vi "New User.vi"() -> ()   [LabVIEW 2020, in "User Lib.lvlib"]
uses:
  User Lib.lvlib
  <vilib>/addons/database/Connection.llb/DB Tools Open Connec (String).vi
  <vilib>/addons/database/_DB Variant To Data/Database Variant To Data.xnode
  <vilib>/addons/database/NI_Database_API.lvlib
  Database Lib.lvlib
panel:
  out "Error out":errorcluster
  out "Error out 2":errorcluster
  in  "Cancel":bool
  in  "OK":bool
  in  "Is Admin?":enum32{"Yes", "No"}(radio)
  in  "Full Name":string
  in  "Confirm Password":string
  in  "Password":string
  in  "Username":string
  # "New User"
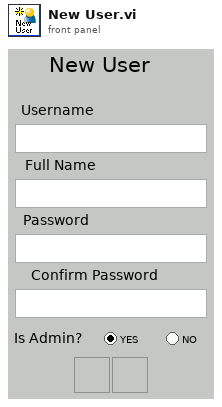
[diagram p1: front panel]
types:
  T1 = cluster{"date/time string":string, "date/time string":string, "code":i32, "date/time string":string, "source":string}
  T2 = typedef "NI_Database_API.lvlib/Conn ObjectReference.ctl" = refnum<k1>
  T3 = cluster{"Username":string, "Full Name":string, "Password":string, string}
  T4 = cluster{i32, "date/time string":string, "date/time string":string, string}
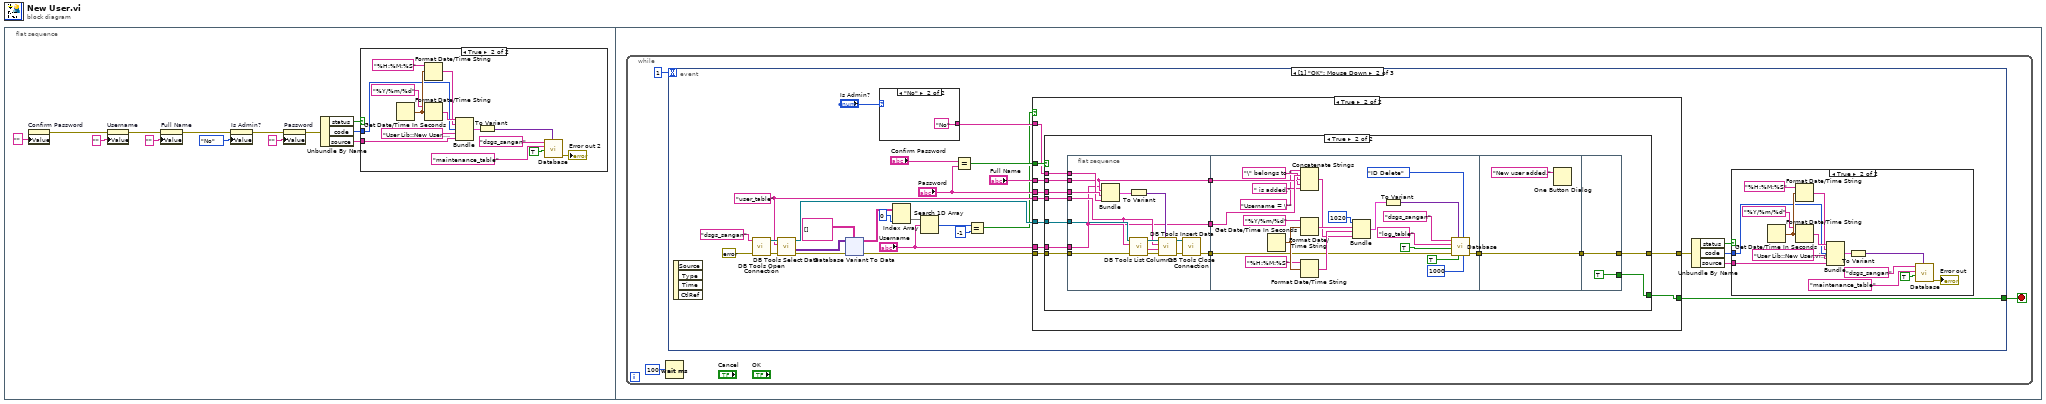
[diagram p0: block diagram]
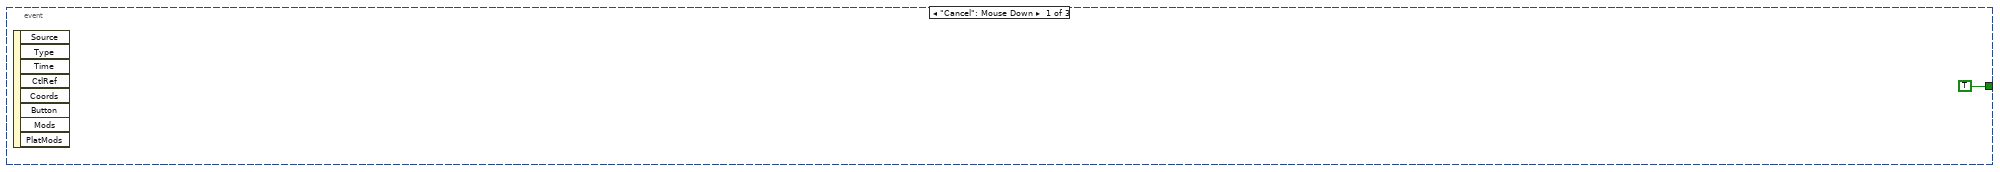
[diagram p3: hidden frame]
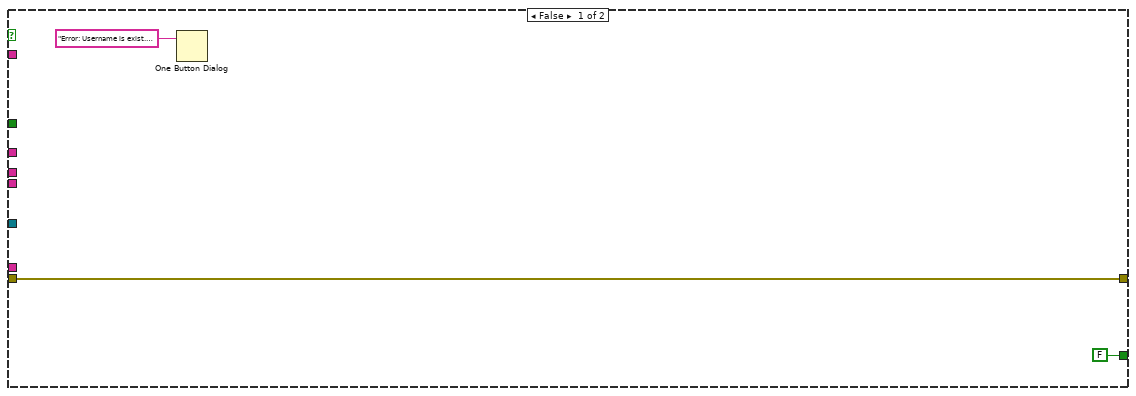
[diagram p5: hidden frame]
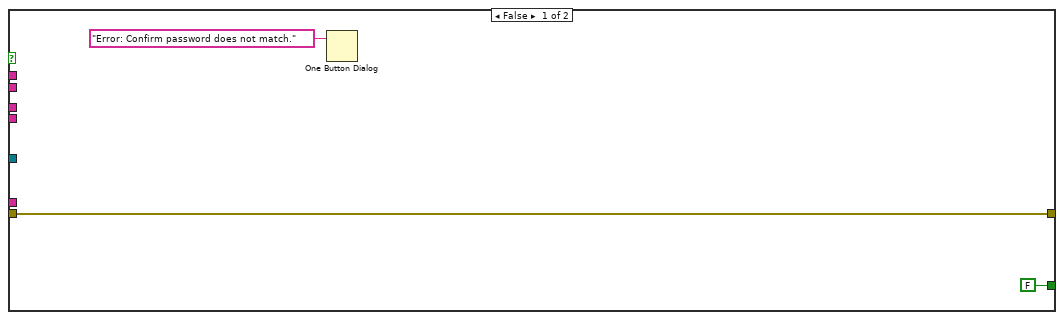
[diagram p6: hidden frame]
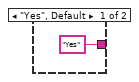
[diagram p7: hidden frame]
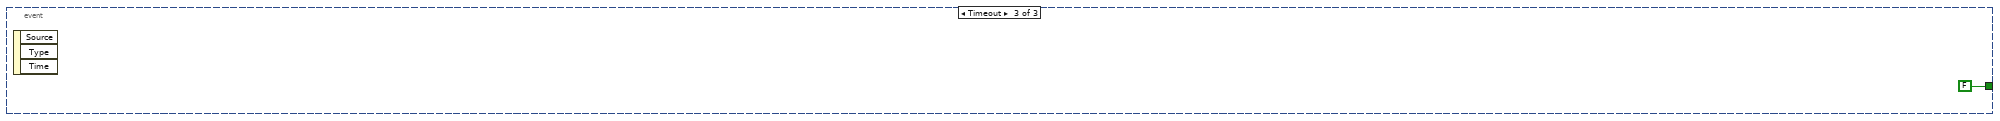
[diagram p8: hidden frame]
diagram:
  n1 = flat-sequence {
    frame #0 {
      n2 = property on="Confirm Password" class="Str"("Value"="" ("Username")) -> (error out=w1:errorcluster)  [unwired: 2 in, 1 out]
      n3 = property on="Username" class="Str"(error in=w1, "Value"="" ("Username")) -> (error out=w2:errorcluster)  [unwired: 1 in, 1 out]
      n4 = property on="Full Name" class="Str"(error in=w2, "Value"="" ("Full Name")) -> (error out=w3:errorcluster)  [unwired: 1 in, 1 out]
      n5 = property on="Is Admin?" class="RadioBtnsControl (strict)"(error in=w3, "Value"=enum32{"Yes", "No"}."No" ("Is Admin?")) -> (error out=w4:errorcluster)  [unwired: 1 in, 1 out]
      n6 = property on="Password" class="Str"(error in=w4, "Value"="" ("Username")) -> (error out=w5:errorcluster)  [unwired: 1 in, 1 out]
      n7 = Unbundle By Name(w5) -> ("status"=w7:bool, "code"=w8:i32, "source"=w6:string)
      n8 = case shown="True" w7 {
        tunnel: w8 -> [_ w22]
        tunnel: w6 -> [_ w20]
        frame False {
        }
        frame True {
          n9 = Get Date/Time In Seconds() -> (seconds since 1Jan1904=w27:timestamp)
          n10 = Format Date/Time String(time format string (%c)="%H:%M:%S", seconds (now)=w27) -> (date/time string=w23:string)  [unwired: 1 in]
          n11 = Format Date/Time String(time format string (%c)="%Y/%m/%d", seconds (now)=w27) -> (date/time string=w24:string)  [unwired: 1 in]
          n12 = Bundle("date/time string"=w24, "date/time string"=w23, "code"=w22, "date/time string"="User Lib::New User.vi::Initialize", "source"=w20) -> (w19:T1)  [unwired: 1 in]
          n13 = To Variant(anything=w19) -> (Variant=w18:variant)
          n14 = call "Database.vi"("Data"=w18, "Auto Increment ID?"=TRUE, "Table"="maintenance_table", "Connection"="dsgs_sangan") -> ("Error out"=→"Error out 2":errorcluster)  [unwired: 7 in]
        }
      }
    }
    frame #1 {
      n15 = while {
        stop <- w29 stop-if-true
        n16 = Wait (ms)(milliseconds to wait=u32 100) -> ()  [unwired: 1 out]
        n17 = event shown="[1] \"OK\": Mouse Down" {
          selector: _ -> [_ _ _]
          dyn-events: _ -> [_ _ _]
          timeout: 1 -> [_ _ _]
          tunnel: [TRUE w53 FALSE] -> w29
          event "Cancel": Mouse Down {
            n18 = event-data() -> ()  [unwired: 1 in, 8 out]
          }
          event "OK": Mouse Down {
            w48 = "user_table" ("Heat Table Name")
            n19 = event-data() -> ()  [unwired: 1 in, 4 out]
            n20 = call-poly <vilib>:"DB Tools Open Connection.vi"("error in (no error)"=errorcluster {"status"=FALSE, "code"=0, "source"=""}, "connection information"="dsgs_sangan" ("Connection Name")) -> ("error out"=w52:errorcluster, "connection reference"=w51:T2)  [unwired: 6 in]
            n21 = call <vilib>:"DB Tools Select Data.vi"("error in (no error)"=w52, "table"=w48, "connection reference"=w51) -> ("error out"=w46:errorcluster, "data"=w47:variant[][], "connection reference out"=w49:T2)  [unwired: 3 in]
            n22 = xnode "Database Variant To Data"("database variant"=w47, "error in (no error)"=w46, "type"=string[][] []) -> ("data"=w43:string[][], "error out"=w45:errorcluster)
            n23 = case shown="\"No\"" "Is Admin?" {
              tunnel: ["Yes" "No"] -> w54
              frame "Yes", Default {
              }
              frame "No" {
              }
            }
            n24 = Index Array(array=w43, index (col)=0 ("disabled index (col)")) -> (element=w41:string[])  [unwired: 1 in]
            n25 = Search 1D Array(1D array=w41, element="Username") -> (index of element=w39:i32)  [unwired: 1 in]
            n26 = Equal?(x="Confirm Password", y="Password") -> (x = y?=w57:bool)
            n27 = Equal?(x=w39, y=-1) -> (x = y?=w37:bool)
            n28 = case shown="True" w37 {
              tunnel: w57 -> [_ w86]
              tunnel: "Full Name" -> [_ w85]
              tunnel: "Password" -> [_ w84]
              tunnel: w54 -> [_ w83]
              tunnel: [FALSE w82] -> w53
              tunnel: w49 -> [_ w81]
              tunnel: [w75 w77] -> w32
              tunnel: w48 -> [_ w80]
              tunnel: w45 -> [w75 w79]
              tunnel: "Username" -> [_ w78]
              frame False {
                n29 = One Button Dialog(message="Error: Username is exist. Please choose another username.") -> ()  [unwired: 1 in, 1 out]
              }
              frame True {
                n30 = case shown="True" w86 {
                  tunnel: w78 -> [_ w103]
                  tunnel: w85 -> [_ w102]
                  tunnel: w84 -> [_ w101]
                  tunnel: w83 -> [_ w100]
                  tunnel: [FALSE w96] -> w82
                  tunnel: w79 -> [w87 w99]
                  tunnel: w81 -> [_ w98]
                  tunnel: [w87 w92] -> w77
                  tunnel: w80 -> [_ w97]
                  frame False {
                    n31 = One Button Dialog(message="Error: Confirm password does not match.") -> ()  [unwired: 1 in, 1 out]
                  }
                  frame True {
                    n32 = flat-sequence {
                      tunnel: w103 -> [w107]
                      tunnel: w102 -> [w108]
                      tunnel: w101 -> [w118]
                      tunnel: w100 -> [w117]
                      tunnel: w99 -> [w112]
                      tunnel: w98 -> [w111]
                      tunnel: w97 -> [w109]
                      tunnel: [w108] -> w95
                      tunnel: [w107] -> w94
                      tunnel: [w105] -> w93
                      tunnel: w95 -> [w126]
                      tunnel: w94 -> [w128]
                      tunnel: w93 -> [w123]
                      tunnel: [w122] -> w90
                      tunnel: [w141] -> w91
                      tunnel: w90 -> [w141]
                      tunnel: [TRUE] -> w96
                      tunnel: [w143] -> w92
                      tunnel: w91 -> [w143]
                      frame #0 {
                        n33 = Bundle("Username"=w107, "Full Name"=w108, "Password"=w118, w117) -> (w113:T3)  [unwired: 1 in]
                        n34 = To Variant(anything=w113) -> (Variant=w116:variant)
                        n35 = call <vilib>:"DB Tools List Columns.vi"("error in (no error)"=w112, "table"=w109, "connection reference"=w111) -> ("error out"=w115:errorcluster, "columns"=w104:string[], "connection reference out"=w114:T2)  [unwired: 1 in, 1 out]
                        n36 = call <vilib>:"DB Tools Insert Data.vi"("data"=w116, "error in (no error)"=w115, "columns"=w104, "table"=w109, "connection reference"=w114) -> ("error out"=w106:errorcluster, "connection reference out"=w110:T2)  [unwired: 5 in]
                        n37 = call <vilib>:"DB Tools Close Connection.vi"("error in (no error)"=w106, "connection reference"=w110) -> ("error out"=w105:errorcluster)  [unwired: 5 in]
                      }
                      frame #1 {
                        n38 = Get Date/Time In Seconds() -> (seconds since 1Jan1904=w136:timestamp)
                        n39 = Concatenate Strings("Username = \"" ("string"), w128, "\" belongs to " ("string"), w126, " is added." ("string")) -> (w124:string)
                        n40 = Format Date/Time String(time format string (%c)="%Y/%m/%d", seconds (now)=w136) -> (date/time string=w137:string)  [unwired: 1 in]
                        n41 = Format Date/Time String(time format string (%c)="%H:%M:%S", seconds (now)=w136) -> (date/time string=w138:string)  [unwired: 1 in]
                        n42 = Bundle(1020, "date/time string"=w137, "date/time string"=w138, w124) -> (w139:T4)  [unwired: 1 in]
                        n43 = To Variant(anything=w139) -> (Variant=w140:variant)
                        n44 = call "Database.vi"("Maximum Row"=1000, "Enum"=enum16{"ID Delete", "Time Delete"}."ID Delete", "Delete row?"=TRUE, "Data"=w140, "Error in"=w123, "Auto Increment ID?"=TRUE, "Table"="log_table" ("table"), "Connection"="dsgs_sangan" ("table")) -> ("Error out"=w122:errorcluster)  [unwired: 3 in]
                      }
                      frame #2 {
                        n45 = One Button Dialog(message="New user added.") -> ()  [unwired: 1 in, 1 out]
                      }
                      frame #3 {
                      }
                    }
                  }
                }
              }
            }
            n46 = Unbundle By Name(w32) -> ("status"=w34:bool, "code"=w35:i32, "source"=w33:string)
            n47 = case shown="True" w34 {
              tunnel: w35 -> [_ w68]
              tunnel: w33 -> [_ w66]
              frame False {
              }
              frame True {
                n48 = Get Date/Time In Seconds() -> (seconds since 1Jan1904=w73:timestamp)
                n49 = Format Date/Time String(time format string (%c)="%H:%M:%S", seconds (now)=w73) -> (date/time string=w69:string)  [unwired: 1 in]
                n50 = Format Date/Time String(time format string (%c)="%Y/%m/%d", seconds (now)=w73) -> (date/time string=w70:string)  [unwired: 1 in]
                n51 = Bundle("date/time string"=w70, "date/time string"=w69, "code"=w68, "date/time string"="User Lib::New User.vi::\"OK\" case", "source"=w66) -> (w65:T1)  [unwired: 1 in]
                n52 = To Variant(anything=w65) -> (Variant=w64:variant)
                n53 = call "Database.vi"("Data"=w64, "Auto Increment ID?"=TRUE, "Table"="maintenance_table", "Connection"="dsgs_sangan") -> ("Error out"=→"Error out":errorcluster)  [unwired: 7 in]
              }
            }
          }
          event Timeout {
            n54 = event-data() -> ()  [unwired: 1 in, 3 out]
          }
        }
      }
    }
  }
